vi "ArmTest_RLE_and_XYZ-AUTO.vi"() -> ()   [LabVIEW 2020]
doc: "Auto test program that coverts RLE to XYZ then to XYZ to RLE"
uses:
  <vilib>/Rock Robotics/WPI/ThirdParty/JAS_Junk/TrajLib/Trajectory_Library.lvlib
panel:
  out "Passed":bool
  out "Extend 2":dbl
  out "Lift 2":dbl
  out "Rotate 2":dbl
  out "z":dbl
  out "y":dbl
  out "x":dbl
  out "Rotate":dbl
  out "Lift":dbl
  out "Extend":dbl
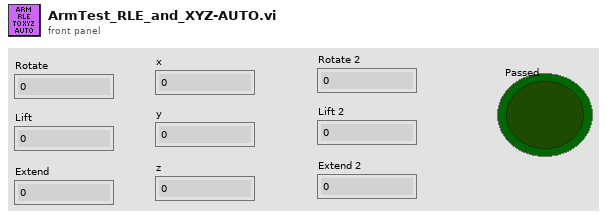
[diagram p1: front panel]
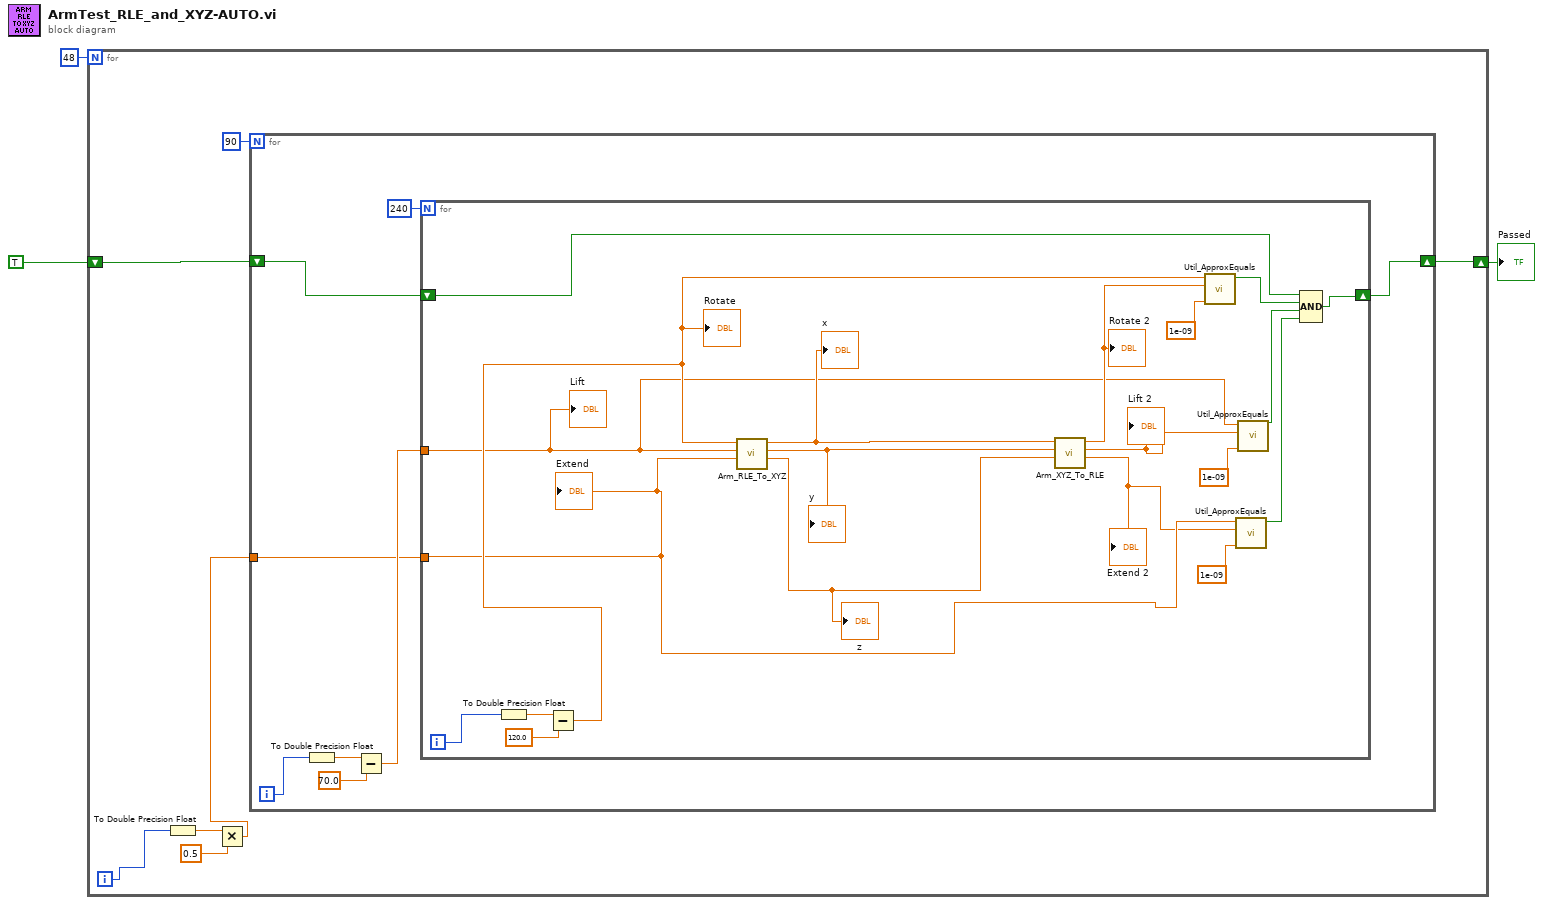
[diagram p0: block diagram]
diagram:
  n1 = for {
    N: 48 -> [_]
    shift-right: [w4] -> w1
    shift-left: TRUE -> [w5]
    i -> [w7]
    n2 = To Double Precision Float(number=w7) -> (double precision float=w9:dbl)
    n3 = Multiply(x=w9, y=0.5) -> (x*y=w6:dbl)
    n4 = for {
      N: 90 -> [_]
      tunnel: w6 -> [w13]
      shift-right: [w11] -> w4
      shift-left: w5 -> [w12]
      i -> [w15]
      n5 = To Double Precision Float(number=w15) -> (double precision float=w17:dbl)
      n6 = Subtract(x=w17, y=70.0) -> (x-y=w14:dbl)
      n7 = for {
        N: 240 -> [_]
        tunnel: w14 -> [w27]
        tunnel: w13 -> [w25]
        shift-right: [w19] -> w11
        shift-left: w12 -> [w23]
        i -> [w35]
        n8 = To Double Precision Float(number=w35) -> (double precision float=w34:dbl)
        n9 = Subtract(x=w34, y=120.0) -> (x-y=w29:dbl)
        "Rotate" <- w29
        n10 = call "Arm_RLE_To_XYZ.vi"("Extend"=w25, "Lift"=w27, "Rotate"=w29) -> ("z"=w36:dbl, "y"=w37:dbl, "x"=w38:dbl)  [unwired: 6 in]
        "x" <- w38
        "y" <- w37
        "z" <- w36
        n11 = call "Arm_XYZ_To_RLE.vi"("Z"=w36, "Y"=w37, "X"=w38) -> ("Extend"=w24:dbl, "Lift"=w26:dbl, "Rotate"=w28:dbl)  [unwired: 6 in]
        "Rotate 2" <- w28
        "Lift 2" <- w26
        "Extend 2" <- w24
        n12 = call <vilib>:"Util_ApproxEquals.vi"("Tolerance"=1e-09, "Value 2"=w28, "Value 1"=w29) -> ("ApproxEquals"=w22:bool)  [unwired: 8 in]
        n13 = call <vilib>:"Util_ApproxEquals.vi"("Tolerance"=1e-09, "Value 2"=w24, "Value 1"=w25) -> ("ApproxEquals"=w20:bool)  [unwired: 8 in]
        n14 = call <vilib>:"Util_ApproxEquals.vi"("Tolerance"=1e-09, "Value 2"=w26, "Value 1"=w27) -> ("ApproxEquals"=w21:bool)  [unwired: 8 in]
        n15 = Compound Arithmetic op=AND(w23, w22, w21, w20) -> (w19:bool)
        "Extend" <- w25
        "Lift" <- w27
      }
    }
  }
  "Passed" <- w1
